vi "PARALLEL FINAL.vi"() -> ()   [LabVIEW 2025]
uses:
  Global 1.vi
  <resource>/objmgr/daqmx.rc
  <vilib>/Analysis/NI_AALBase.lvlib
  <vilib>/DAQmx/read.llb/DAQmx Read (Analog 1D DBL 1Chan NSamp).vi
  <vilib>/DAQmx/create/channels.llb/DAQmx Create Channel (AI-Voltage-Basic).vi
  <vilib>/DAQmx/configure/timing.llb/DAQmx Timing (Sample Clock).vi
  <vilib>/Analysis/1siggen.llb/Ramp Pattern by Samples.vi
  <vilib>/Utility/file.llb/Write To Spreadsheet File (DBL).vi
panel:
  in  "?":bool
  out "Total time of acquisition [s]":dbl
  out "Graphe XY":cluster{dbl[], dbl[]}[](graph)
  out "N":dbl=1000.0 format="%0.2f"
  out "T":dbl
  out "dt":dbl
  out "x < 0?":bool
  in  "Stop":bool
  in  "File path":path
  in  "Channel":string(combo)="/ai0"
  in  "Sampling frecuency [Hz]":dbl=1000.0 format="%0.2f"
  # "HEART RATE VARIABILITY ESTIMATORS FOR STRESS DETECTION"
  # "ECG acquisition in real time"
  # "MARCON Pietro, MAZZANTE Lorenzo, SCORZA Martín"
  # "BM04 -Université de technologie de Compiègne"
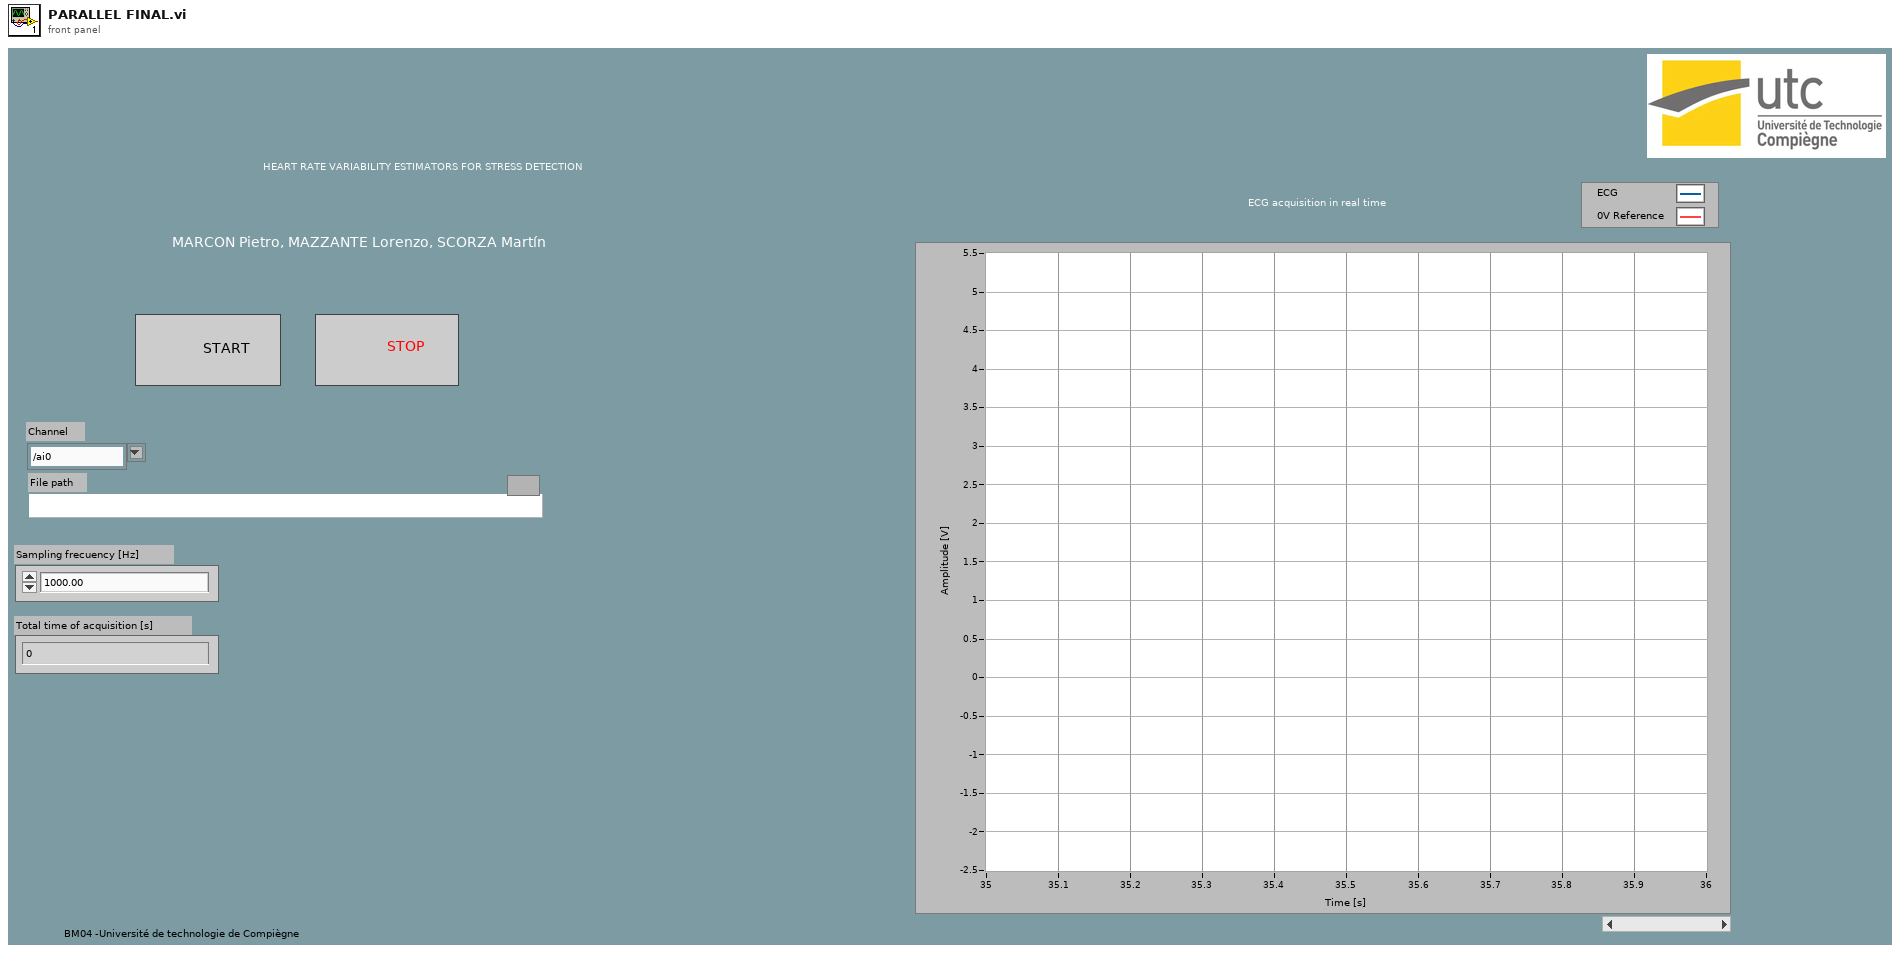
[diagram p1: front panel]
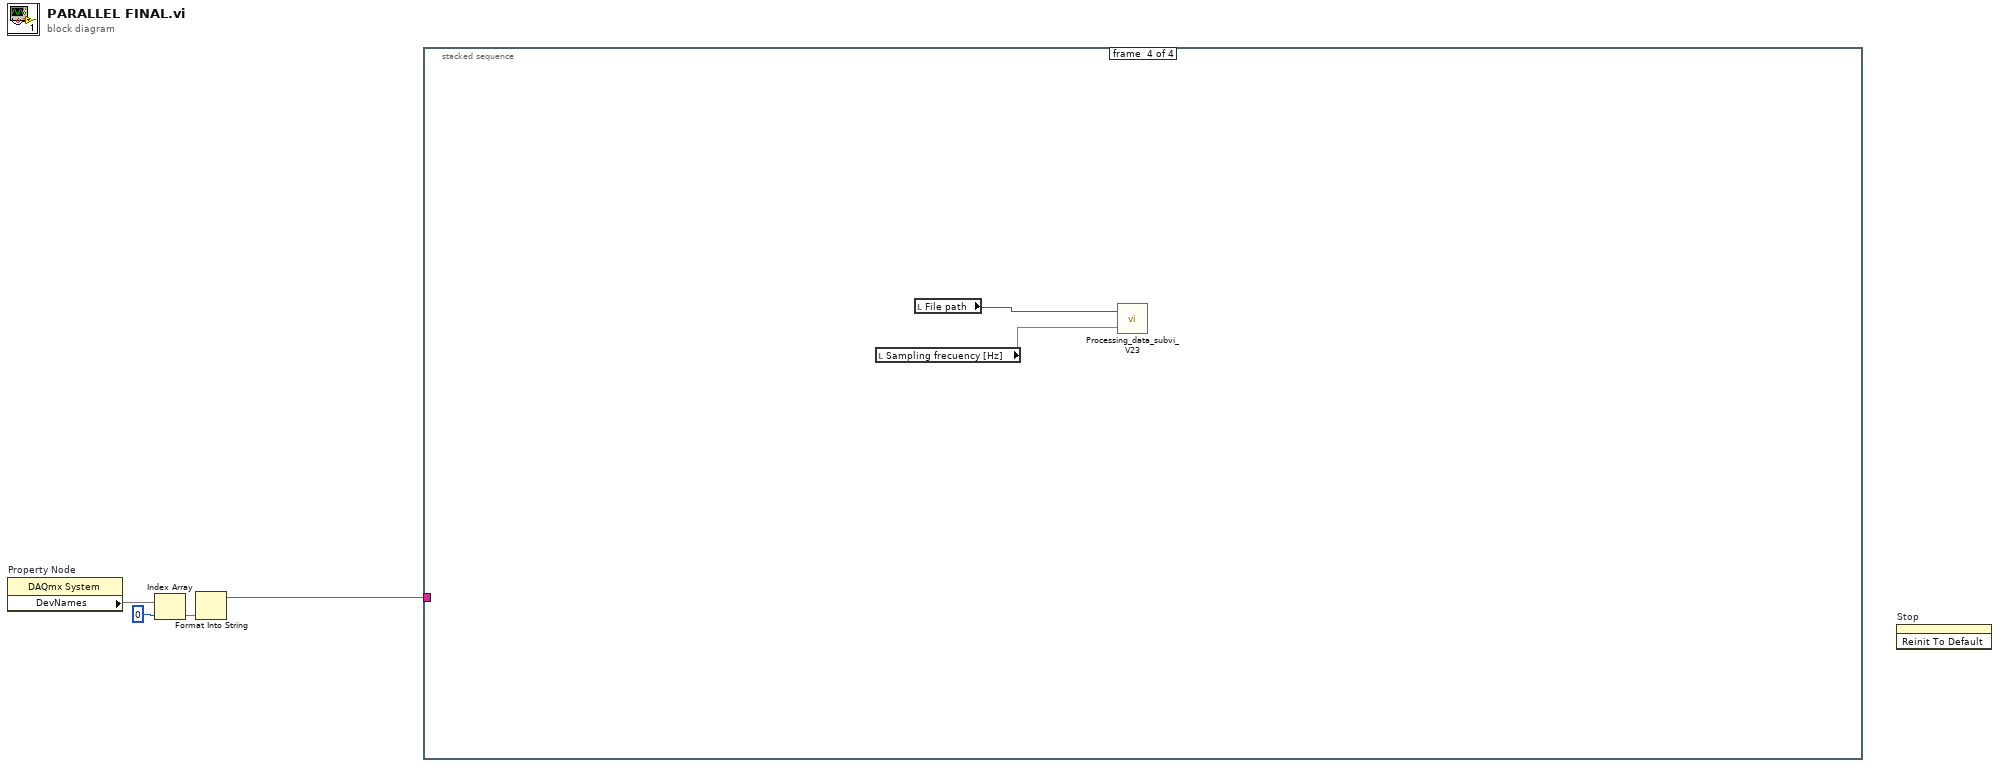
[diagram p0: block diagram]
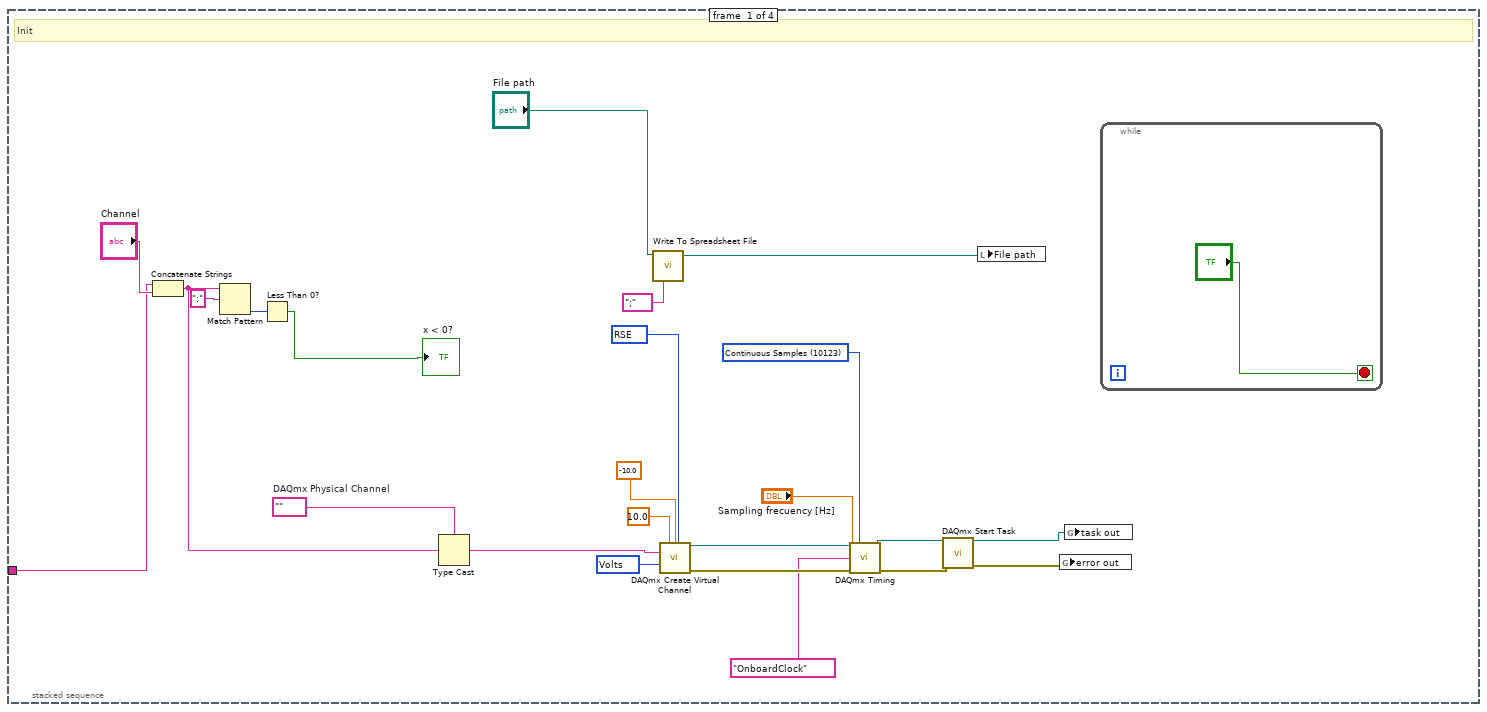
[diagram p2: hidden frame]
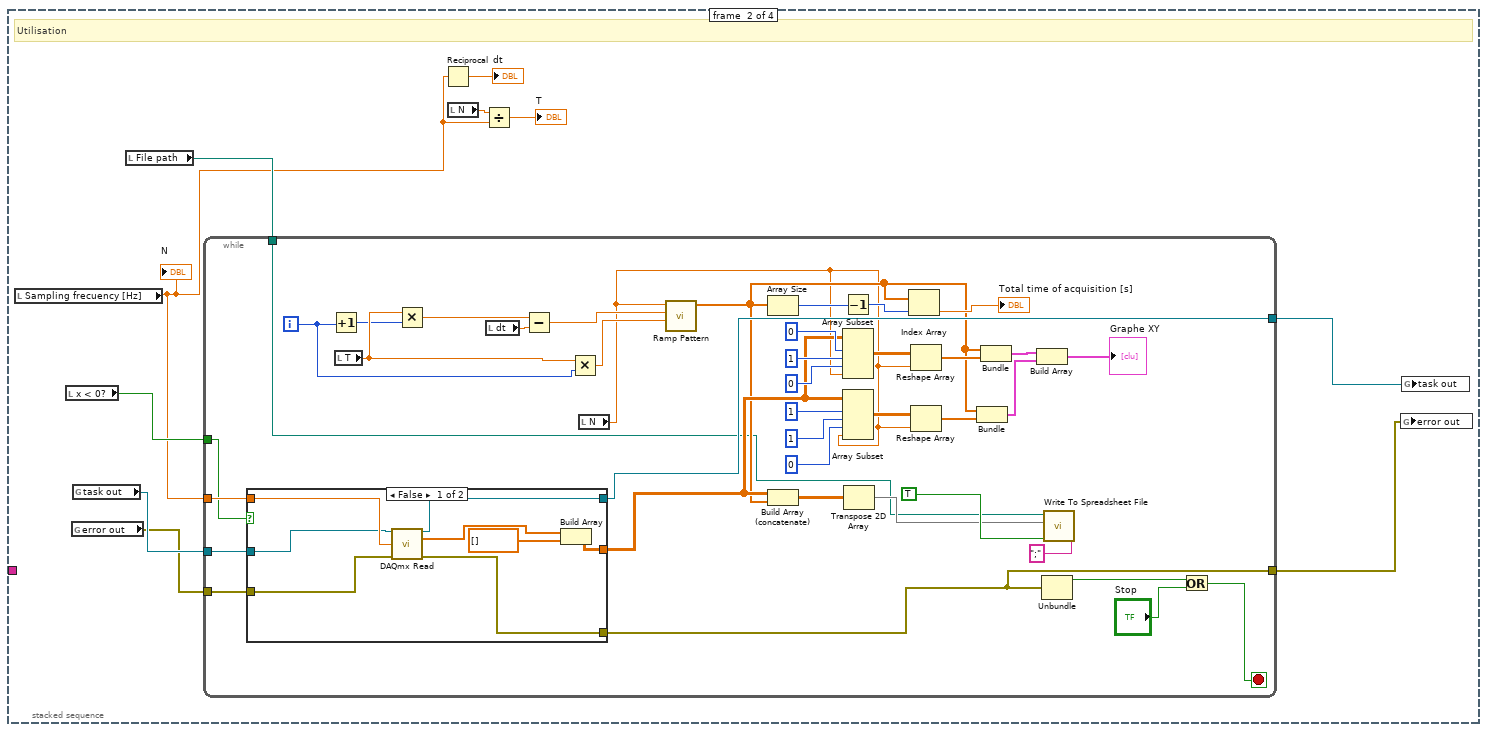
[diagram p3: hidden frame]
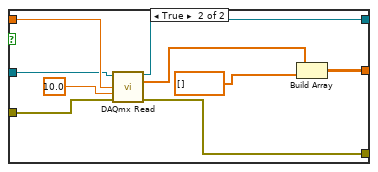
[diagram p4: hidden frame]
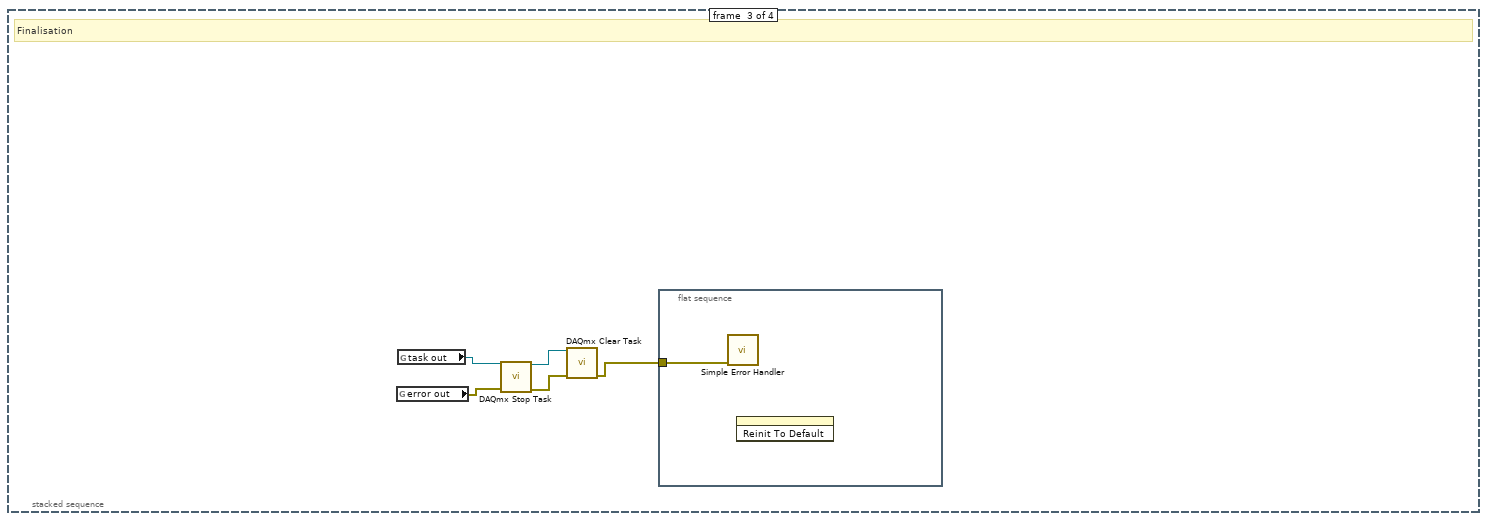
[diagram p5: hidden frame]
diagram:
  n1 = property on="Property Node" class="DAQmx System"() -> ("DevNames"=w4)  [unwired: 2 in, 2 out]
  n2 = Index Array "Index Array"(array=w4, index=0) -> (element=w2)
  n3 = Format Into String "Format Into String"(w2) -> (resulting string=w1:string)  [unwired: 3 in, 1 out]
  n4 = stacked-sequence {
    tunnel: w1 -> [w9 _ _ _]
    frame #0 {
      w7 = tag ""  # DAQmx Physical Channel
      w20 = 10123 items=["Finite Samples"=10178, "Continuous Samples"=10123, "Hardware Timed Single Point"=12522] ("sample mode")
      w25 = 10083 items=["Default"=-1, "RSE"=10083, "NRSE"=10078, "Differential"=10106, "Pseudodifferential"=12529] ("input terminal configuration")
      w26 = 10348 items=["Volts"=10348, "From Custom Scale"=10065] ("units")
      # "Init"
      n5 = Concatenate Strings "Concatenate Strings"(w9, "Channel") -> (w10:string)
      n6 = Match Pattern(string=w10, regular expression=":") -> (offset past match=w13:i32)  [unwired: 1 in, 3 out]
      n7 = Less Than 0?(x=w13) -> (x < 0?=→"x < 0?":bool)
      n8 = Type Cast(type=w7, x=w10) -> (*(type *) &x=w12:tag)
      n9 = call-poly <vilib>:"Write To Spreadsheet File.vi"("delimiter (\\t)"=";" ("delimiter (\\t)"), "file path (dialog if empty)"="File path") -> ("new file path (Not A Path if cancelled)"=w6:path)  [unwired: 6 in]
      n10 = call-poly <vilib>:"DAQmx Create Virtual Channel.vi"("maximum value"=10.0, "minimum value"=-10.0, "input terminal configuration"=w25, "physical channels"=w12, "units"=w26) -> ("task out"=w24:refnum<k21>, "error out"=w23:errorcluster)  [unwired: 9 in]
      n11 = call-poly <vilib>:"DAQmx Timing.vi"("task/channels in"=w24, "sample mode"=w20, "rate"="Sampling frecuency [Hz]", "source"=tag "OnboardClock", "error in"=w23) -> ("task out"=w19:refnum<k21>, "error out"=w18:errorcluster)  [unwired: 9 in]
      n12 = call <vilib>:"DAQmx Start Task.vi"("task/channels in"=w19, "error in"=w18) -> ("task out"=w16:refnum<k21>, "error out"=w17:errorcluster)  [unwired: 12 in]
      n13 = local write "File path"(w6) -> ()
      n14 = global write "Global 1.vi" "error out"(w17) -> ()
      n15 = global write "Global 1.vi" "task out"(w16) -> ()
      n16 = while {
        stop <- "?" stop-if-true
      }
    }
    frame #1 {
      # "Utilisation"
      n17 = local read "Sampling frecuency [Hz]"() -> (w32:dbl)
      "N" <- w32
      n18 = local read "x < 0?"() -> (w36:bool)
      n19 = global read "Global 1.vi" "error out"() -> (w38:errorcluster)
      n20 = global read "Global 1.vi" "task out"() -> (w39:refnum<k21>)
      n21 = local read "File path"() -> (w37:path)
      n22 = while {
        tunnel: w32 -> [w79]
        tunnel: w39 -> [w78]
        tunnel: w38 -> [w77]
        tunnel: w36 -> [w73]
        tunnel: w37 -> [w50]
        tunnel: [w52] -> w31
        tunnel: [w49] -> w30
        i -> [w44]
        stop <- w74 stop-if-true
        n23 = case shown="False" w73 {
          tunnel: w79 -> [w85 w93]
          tunnel: w78 -> [w84 w92]
          tunnel: w77 -> [w83 w91]
          tunnel: [w81 w90] -> w52
          tunnel: [w82 w89] -> w49
          tunnel: [w80 w88] -> w53
          frame False {
            n24 = call-poly <vilib>:"DAQmx Read.vi"("task/channels in"=w84, "number of samples per channel"=w85, "error in"=w83) -> ("task out"=w81:refnum<k21>, "data"=w86:dbl[], "error out"=w82:errorcluster)  [unwired: 10 in]
            n25 = Build Array(w86, dbl[] []) -> (w80:dbl[][])
          }
          frame True {
            n26 = call-poly <vilib>:"DAQmx Read.vi"("task/channels in"=w92, "number of samples per channel"=w93, "timeout"=10.0, "error in"=w91) -> ("task out"=w90:refnum<k21>, "data"=w95:dbl[], "error out"=w89:errorcluster)  [unwired: 9 in]
            n27 = Build Array(w95, dbl[] []) -> (w88:dbl[][])
          }
        }
        n28 = Increment(x=w44) -> (x+1=w45:i32)
        n29 = local read "T"() -> (w46:dbl)
        n30 = Multiply(x=w46, y=w45) -> (x*y=w47:dbl)
        n31 = local read "dt"() -> (w48:dbl)
        n32 = Subtract(x=w47, y=w48) -> (x-y=w42:dbl)
        n33 = Multiply(x=w46, y=w44) -> (x*y=w43:dbl)
        n34 = local read "N"() -> (w41:dbl)
        n35 = call-poly <vilib>:"Ramp Pattern.vi"("start"=w43, "end"=w42, "samples"=w41) -> ("Ramp Pattern"=w51:dbl[])  [unwired: 7 in, 1 out]
        n36 = Array Size(array=w51) -> (size(s)=w58:i32)
        n37 = Build Array (concatenate)(w53, w51) -> (w59:dbl[][])
        n38 = Decrement(x=w58) -> (x-1=w56:i32)
        n39 = Array Subset(array=w53, index (row)=0, length (row)=1, index (col)=0, length (col)=w41) -> (w61:dbl[][])
        n40 = Array Subset(array=w53, index (row)=1, length (row)=1, index (col)=0, length (col)=w41) -> (w63:dbl[][])
        n41 = Transpose 2D Array(2D array=w59) -> (transposed array=w71:dbl[][])
        n42 = Index Array(array=w51, index=w56) -> (element=→"Total time of acquisition [s]":dbl)
        n43 = Reshape Array(w61, w41) -> (w60:dbl[])
        n44 = Reshape Array(w63, w41) -> (w62:dbl[])
        n45 = Bundle("Ramp Pattern"=w51, w62) -> (w54:cluster{"Ramp Pattern":dbl[], dbl[]})  [unwired: 1 in]
        n46 = Bundle("Ramp Pattern"=w51, w60) -> (w55:cluster{"Ramp Pattern":dbl[], dbl[]})  [unwired: 1 in]
        n47 = Build Array(w55, w54) -> (→"Graphe XY":cluster{"Ramp Pattern":dbl[], dbl[]}[])
        n48 = Unbundle(w49) -> ("status"=w75:bool)  [unwired: 2 out]
        n49 = call-poly <vilib>:"Write To Spreadsheet File.vi"("delimiter (\\t)"=";" ("delimiter (\\t)"), "append to file? (new file:F)"=TRUE, "2D data"=w71, "file path (dialog if empty)"=w50) -> ()  [unwired: 4 in, 1 out]
        n50 = Or(x=w75, y="Stop") -> (x .or. y?=w74:bool)
      }
      n51 = Reciprocal(x=w32) -> (1/x=→"dt":dbl)
      n52 = local read "N"() -> (w34:dbl)
      n53 = Divide(x=w34, y=w32) -> (x/y=→"T":dbl)
      n54 = global write "Global 1.vi" "error out"(w30) -> ()
      n55 = global write "Global 1.vi" "task out"(w31) -> ()
    }
    frame #2 {
      # "Finalisation"
      n56 = global read "Global 1.vi" "error out"() -> (w98:errorcluster)
      n57 = global read "Global 1.vi" "task out"() -> (w99:refnum<k21>)
      n58 = call <vilib>:"DAQmx Stop Task.vi"("task/channels in"=w99, "error in"=w98) -> ("task out"=w101:refnum<k21>, "error out"=w100:errorcluster)  [unwired: 12 in]
      n59 = call <vilib>:"DAQmx Clear Task.vi"("task in"=w101, "error in"=w100) -> ("error out"=w97:errorcluster)  [unwired: 13 in]
      n60 = flat-sequence {
        tunnel: w97 -> [w102]
        frame #0 {
          n61 = call <vilib>:"Simple Error Handler.vi"("error in (no error)"=w102) -> ()  [unwired: 4 in, 5 out]
          n62 = invoke class="Bool" method="Reinit To Default"() -> ()  [unwired: 3 in, 3 out]
        }
      }
    }
    frame #3 {
      n63 = local read "Sampling frecuency [Hz]"() -> (w103:dbl)
      n64 = local read "File path"() -> (w104:path)
      n65 = call "Processing_data_subvi_V23.vi"("Sampling Frecuency [Hz]"=w103, "file path (use dialog)"=w104) -> ()  [unwired: 2 out]
    }
  }
  n66 = invoke on="Stop" class="Bool" method="Reinit To Default"() -> ()  [unwired: 3 in, 3 out]
